vi "LKIF2_GetCalcData.vi"(7 "OutNo (OUT1)":T1=1 items=["OUT01"=1, "OUT02"=2, "OUT03"=4, "OUT04"=8, "OUT05"=16, "OUT06"=32, "OUT07"=64, "OUT08"=128, "OUT09"=256, "OUT10"=512, "OUT11"=1024, "OUT12"=2048, "ALL OUT"=4095], 8 "error in (no error)":errorcluster {"code" format="%x"}, 11 "path in":path) -> (0 "error out":errorcluster {"code" format="%x"}, 3 "CalcData":T3(array[cluster]) {"LKIF_FLOATRESULT" items=["VALID", "RANGEOVER_P", "RANGEOVER_N", "WAITING", "ALARM", "INVALID"]})   [LabVIEW 2014, in "Keyence LK-G5000.lvlib"]
uses:
  <instrlib>/Keyence LK-G5000/Keyence LK-G5000.lvlib
  <instrlib>/Keyence LK-G5000/Public/enum/LKIF_FLOATRESULT.ctl
  <instrlib>/Keyence LK-G5000/Public/enum/LKIF_OUTNO.ctl
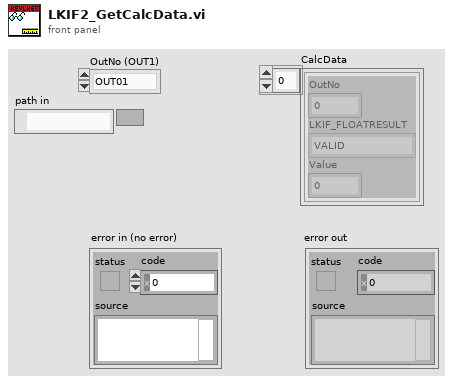
[diagram p1: front panel]
types:
  T1 = typedef "Keyence LK-G5000.lvlib/LKIF_OUTNO.ctl" = i32
  T2 = typedef "Keyence LK-G5000.lvlib/LKIF_FLOATRESULT.ctl" = i32
  T3 = cluster{"OutNo":i32, "LKIF_FLOATRESULT":T2, "Value":sgl}[]
  T4 = cluster{"OutNo":i32, "LKIF_FLOATRESULT":T2, "Value":sgl}
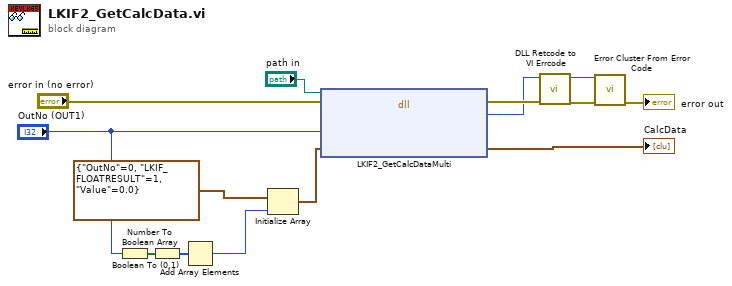
[diagram p0: block diagram]
diagram:
  n1 = Number To Boolean Array(number="OutNo (OUT1)") -> (Boolean array=w11:bool[])
  n2 = Boolean To (0,1)(Boolean=w11) -> (0, 1=w10:i16[])
  n3 = Add Array Elements(numeric array=w10) -> (sum=w8:i16)
  n4 = Initialize Array(T4 {"OutNo"=0, "LKIF_FLOATRESULT"=1, "Value"=0.0} ("LKIF_FLOATVALUE_OUT"), w8) -> (w7:T3)
  n5 = dll-call lib="C:/Program Files/National Instruments/LabVIEW 2011/instr.lib/Keyence LK-G5000/LKIF2.dll" fn="LKIF2_GetCalcDataMulti"(path in="path in", error in="error in (no error)", "OutNo"="OutNo (OUT1)", "CalcData"=w7) -> (error out=w6:errorcluster, "RC"=w5:i32, "CalcData"=→"CalcData":T3)  [unwired: 2 in, 1 out]
  n6 = call <instrlib>:"DLL Retcode to VI Errcode.vi"("error in (no error)"=w6, "DLL Retcode"=w5) -> ("error out"=w14:errorcluster, "VI Errcode"=w13:i32)  [unwired: 8 in]
  n7 = call <vilib>:"Error Cluster From Error Code.vi"("error in (no error)"=w14, "error code (0)"=w13) -> ("error out"=→"error out":errorcluster)  [unwired: 7 in]
